vi "AutoLin Messwert aus Rohwert.vi"(8 "Polynomkoeff.":dbl[](array[numeric]), 11 "Rohwert (ppm)":dbl) -> (3 "Messwert (ppm) linearisiert":dbl)   [LabVIEW 2020, in "Linearisierung v2.lvlib"]
doc: "Muster für Linearisierung der rohen Messwerte mit Hilfe des Linearisierungs-Polynoms, das vom VI \"AutoLin Anpassung\" geliefert wird."
uses:
  Linearisierung v2.lvlib
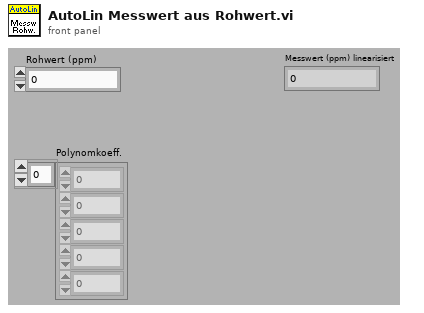
[diagram p1: front panel]
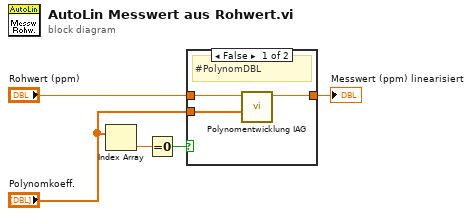
[diagram p0: block diagram]
diagram:
  n1 = Index Array(array="Polynomkoeff.") -> (element=w2:dbl)  [unwired: 1 in]
  n2 = Equal To 0?(x=w2) -> (x = 0?=w1:bool)
  n3 = case shown="False" w1 {
    tunnel: "Rohwert (ppm)" -> [w7 w9]
    tunnel: [w6 w9] -> w4
    tunnel: "Polynomkoeff." -> [w8 _]
    frame False {
      # "#PolynomDBL"
      n4 = call "Polynomentwicklung IAG.vi"("P(x)"=w8, "a"=w7) -> ("P(a)"=w6:dbl)  [unwired: 9 in]
    }
    frame True {
    }
  }
  "Messwert (ppm) linearisiert" <- w4
